vi "Create ICS.vi"(7 "Messenger":refnum<class "Messenger.lvclass">, 8 "error in (no error)":errorcluster, 9 "motors":refnum<class "Motor.lvclass">[](array[class]), 10 "control indices":i32[](array[numeric]), 11 "email settings":T1) -> (0 "error out":errorcluster, 3 "ICS out":refnum<class "ICS.lvclass">)   [LabVIEW 2018, in "ICS.lvclass"]
uses:
  ICS.lvclass
  Motor/Motor.lvclass
  Messenger/Messenger.lvclass
  TCP-Server/TCP-Server.lvclass
  StateManager/StateManager.lvclass
  MotorManager/MotorManager.lvclass
  C:/Dados/SPARC4/Automacao 2022/S4ICS/StateManager/StateManager.lvclass
  StateManager/StateManager.lvclass/StateManager.ctl
  TCP-Server/TCP-Server.lvclass/TCP-Server.ctl
  ICS.lvclass/ICS.ctl
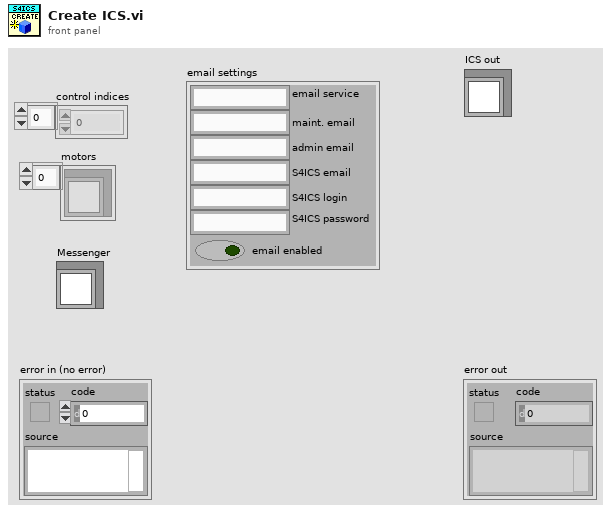
[diagram p1: front panel]
types:
  T1 = cluster{"email service":string, "maint. email":string, "admin email":string, "S4ICS email":string, "S4ICS login":string, "S4ICS password":string, "email enabled":bool}
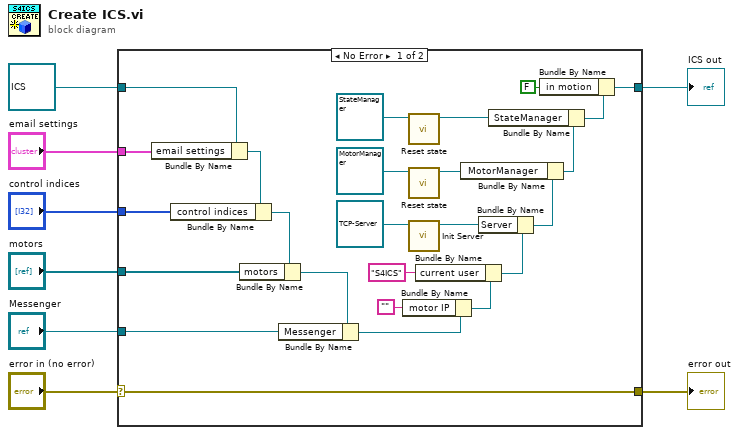
[diagram p0: block diagram]
diagram:
  n1 = case shown="No Error" "error in (no error)" {
    selector: "error in (no error)" -> [w33 w35]
    tunnel: [w33 w35] -> w7
    tunnel: [w20 w34] -> w5
    tunnel: refnum<class "ICS.lvclass"> refnum ("ICS in") -> [w21 w34]
    tunnel: "motors" -> [w27 _]
    tunnel: "email settings" -> [w26 _]
    tunnel: "control indices" -> [w24 _]
    tunnel: "Messenger" -> [w14 _]
    frame No Error {
      n2 = Bundle By Name(cluster=w21, "email settings"=w26) -> (w25:refnum<class "ICS.lvclass">)
      n3 = Bundle By Name(cluster=w25, "control indices"=w24) -> (w23:refnum<class "ICS.lvclass">)
      n4 = Bundle By Name(cluster=w23, "motors"=w27) -> (w16:refnum<class "ICS.lvclass">)
      n5 = Bundle By Name(cluster=w16, "Messenger"=w14) -> (w15:refnum<class "ICS.lvclass">)
      n6 = Bundle By Name(cluster=w15, "motor IP"="") -> (w18:refnum<class "ICS.lvclass">)
      n7 = call "Reset state.vi"("StateManager in"=refnum<class "StateManager.lvclass"> refnum ("StateManager.lvclass")) -> ("StateManager out"=w11:refnum<class "StateManager.lvclass">)  [unwired: 9 in, 1 out]
      n8 = call "Reset state.vi"("StateManager in"=refnum<class "MotorManager.lvclass"> refnum ("MotorManager.lvclass")) -> ("StateManager out"=w9:refnum<class "MotorManager.lvclass">)  [unwired: 9 in, 1 out]
      n9 = call "Init Server.vi"("Server in"=refnum<class "TCP-Server.lvclass"> refnum ("Server.lvclass")) -> ("Server out"=w28:refnum<class "TCP-Server.lvclass">)  [unwired: 9 in, 1 out]
      n10 = Bundle By Name(cluster=w18, "current user"="S4ICS") -> (w22:refnum<class "ICS.lvclass">)
      n11 = Bundle By Name(cluster=w22, "Server"=w28) -> (w13:refnum<class "ICS.lvclass">)
      n12 = Bundle By Name(cluster=w13, "MotorManager"=w9) -> (w12:refnum<class "ICS.lvclass">)
      n13 = Bundle By Name(cluster=w12, "StateManager"=w11) -> (w19:refnum<class "ICS.lvclass">)
      n14 = Bundle By Name(cluster=w19, "in motion"=FALSE) -> (w20:refnum<class "ICS.lvclass">)
    }
    frame Error {
    }
  }
  "error out" <- w7
  "ICS out" <- w5
